vi "GET_Operators_BasicInfo.vi"(7 "Database Ref In":T1, 8 "error in (no error)":errorcluster) -> (0 "error out":errorcluster, 2 "Basic Info":T2[](array[typedef]), 5 "Database Ref Out":T1)   [LabVIEW 2018, in "MySQLTools.lvlib"]
doc: "Returns entryies from Operators table in ostepdb database. If there is no Reference provided, this VI will open a new connection and pass as output."
uses:
  MySQLTools.lvlib
  TypeDefs/BasicOperatorInfo.ctl
  <vilib>/addons/database/Connection.llb/Conn ObjectReference.ctl
  <vilib>/addons/database/NI_Database_API.lvlib
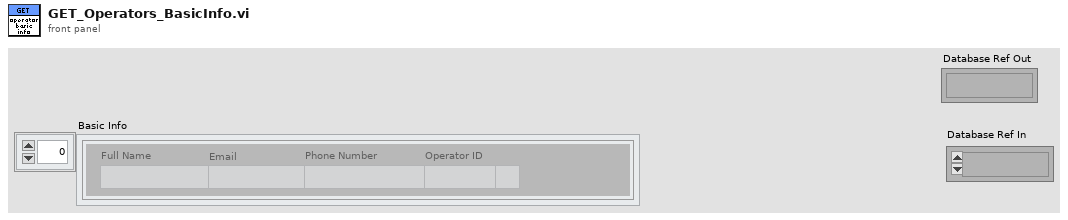
[diagram p1: front panel]
types:
  T1 = typedef "NI_Database_API.lvlib/Conn ObjectReference.ctl" = refnum<k1>
  T2 = typedef "MySQLTools.lvlib/BasicOperatorInfo.ctl" = cluster{"Full Name":string, "Email":string, "Phone Number":string, "Operator ID":string}
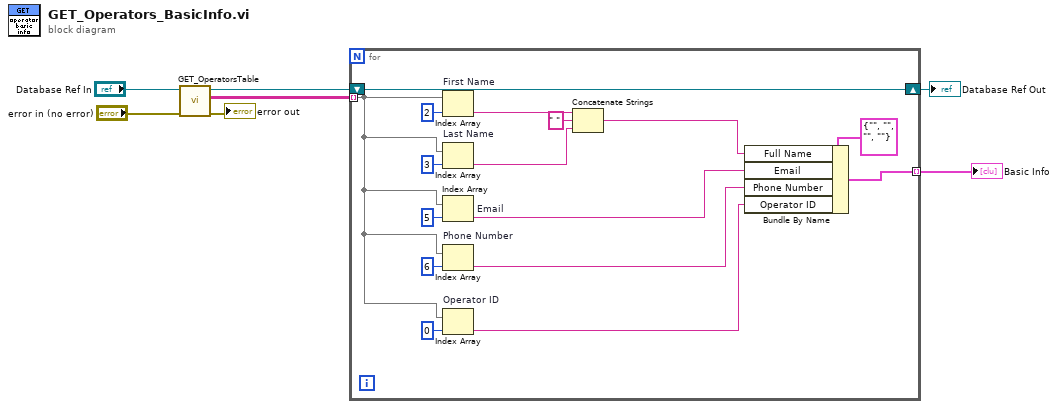
[diagram p0: block diagram]
diagram:
  n1 = call "GET_OperatorsTable.vi"("error in (no error)"="error in (no error)", "Database Ref In"="Database Ref In") -> ("error out"=→"error out":errorcluster, "Array"=w4:string[][], "Database Ref Out"=w3:T1)  [unwired: 7 in]
  n2 = for {
    tunnel: w4 -> [w9] mode=indexing
    tunnel: [w13] -> w6 mode=indexing
    shift-right: [w11] -> w2
    shift-left: w3 -> [w11]
    n3 = Index Array "First Name"(array=w9, index=2) -> (element=w21:string)
    n4 = Index Array "Last Name"(array=w9, index=3) -> (element=w20:string)
    n5 = Index Array "Email"(array=w9, index=5) -> (element=w15:string)
    n6 = Index Array "Phone Number"(array=w9, index=6) -> (element=w14:string)
    n7 = Index Array "Operator ID"(array=w9, index=0) -> (element=w8:string)
    n8 = Concatenate Strings(w21, " " ("string"), w20) -> (w16:string)
    n9 = Bundle By Name(cluster=T2 {"Full Name"="", "Email"="", "Phone Number"="", "Operator ID"=""} ("Basic Info"), "Full Name"=w16, "Email"=w15, "Phone Number"=w14, "Operator ID"=w8) -> (w13:T2)
  }
  "Basic Info" <- w6
  "Database Ref Out" <- w2
